vi "Snake Display.vi"(7 "Color":u32(colorbox), 8 "error in (no error)":errorcluster, 9 "Particle Size":u32, 10 "2D Picture":picture, 11 "Snake in":refnum<class "Snake.lvclass">) -> (0 "error out":errorcluster, 2 "2D Picture Out":picture, 3 "Snake out":refnum<class "Snake.lvclass">)   [LabVIEW 2019, in "Snake.lvclass"]
uses:
  Snake.lvclass
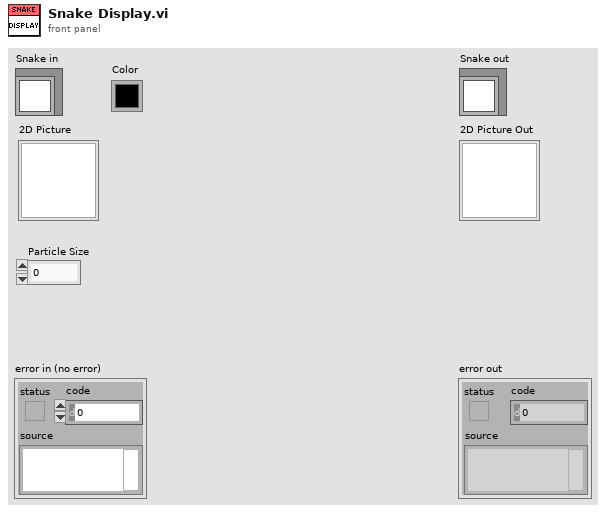
[diagram p1: front panel]
types:
  T1 = typedef "Snake.lvclass/Snake Component STYP.ctl" = cluster{"Direction":T2, "Coordinate":T3}
  T2 = typedef "Direction STYP.ctl" = enum16{"Up", "Down", "Left", "Right"}
  T3 = typedef "Coordinate STYP.ctl" = cluster{"X":i32, "Y":i32}
  T4 = cluster{"left":i16, "top":i16, "right":i16, "bottom":i16}
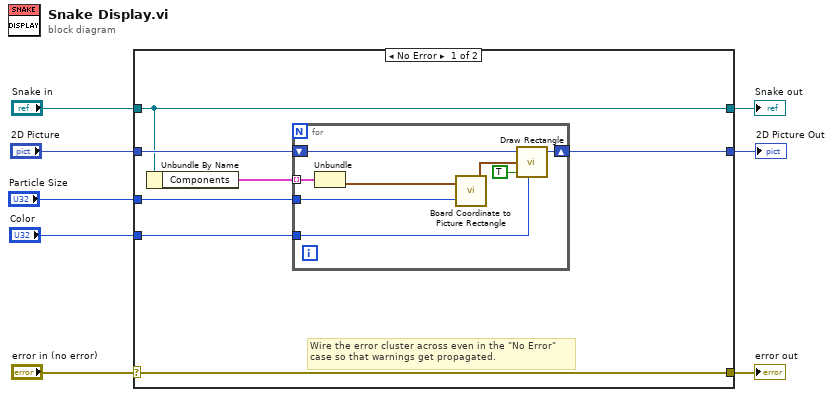
[diagram p0: block diagram]
diagram:
  n1 = case shown="No Error" "error in (no error)" {
    selector: "error in (no error)" -> [w15 w25]
    tunnel: [w15 w25] -> w7
    tunnel: [w11 w24] -> w5
    tunnel: "Snake in" -> [w11 w24]
    tunnel: "2D Picture" -> [w14 _]
    tunnel: "Color" -> [w13 _]
    tunnel: "Particle Size" -> [w12 _]
    tunnel: [w9 _] -> w1
    frame No Error {
      # "Wire the error cluster across even in the \"No Error\"\ncase so that warnings get propagated."
      n2 = Unbundle By Name(w11) -> ("Components"=w10:T1[])
      n3 = for {
        shift-right: [w22] -> w9
        shift-left: w14 -> [w23]
        tunnel: w13 -> [w19]
        tunnel: w12 -> [w18]
        tunnel: w10 -> [w17] mode=indexing
        n4 = Unbundle(w17) -> ("Coordinate"=w16:T3)  [unwired: 1 out]
        n5 = call "Board Coordinate to Picture Rectangle.vi"("Particle Size"=w18, "Coordinate"=w16) -> ("rect"=w21:T4)
        n6 = call <vilib>:"Draw Rectangle.vi"("picture"=w23, "rect"=w21, "fill?(F)"=TRUE, "color(black)"=w19) -> ("new picture"=w22:picture)  [unwired: 5 in]
      }
    }
    frame Error {
    }
  }
  "error out" <- w7
  "Snake out" <- w5
  "2D Picture Out" <- w1
